vi "clone.vi"(0 "reference":refnum<class "SegmentedLineEdge.lvclass">, 5 "error in (no error)":errorcluster) -> (14 "reference out":refnum<class "SegmentedLineEdge.lvclass">, 15 "clonedEdge":refnum<class "AbstractEdge.lvclass">, 19 "error out":errorcluster)   [LabVIEW 2020, in "SegmentedLineEdge.lvclass"]
doc: "clone"
uses:
  <resource>/Framework/Providers/Open_GDS/UML/SegmentedLineEdge_class/SegmentedLineEdge.lvclass
  C:/Program Files (x86)/National Instruments/LabVIEW 2020/resource/Framework/Providers/Open_GDS/UML/GeneralPathEdge_class/GeneralPathEdge.lvclass
  C:/Program Files (x86)/National Instruments/LabVIEW 2020/resource/Framework/Providers/Open_GDS/UML/AbstractEdge_class/AbstractEdge.lvclass
  <resource>/Framework/Providers/Open_GDS/UML/AbstractEdge_class/AbstractEdge.lvclass
  <resource>/Framework/Providers/Open_GDS/UML/GeneralPathEdge_class/GeneralPathEdge.lvclass
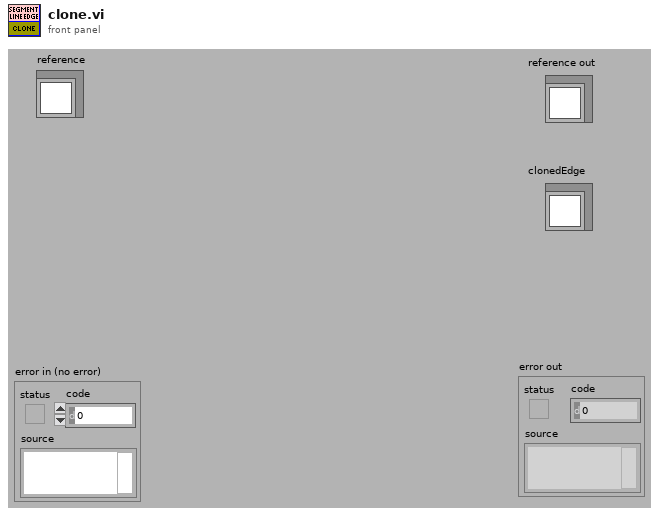
[diagram p1: front panel]
types:
  T1 = typedef "SegmentedLineEdge.lvclass/ObjectAttributes.ctl" = cluster{"lineStyle":refnum<class "LineStyle.lvclass">, "startArrowHead":refnum<class "ArrowHead.lvclass">, "endArrowHead":refnum<class "ArrowHead.lvclass">, "startLabel":string, "midLabel":string, "endLabel":string, "MidLabelOffset":T2, "SplitWire":bool}
  T2 = typedef "Point Point2D.ctl" = cluster{"x":dbl, "y":dbl}
  T3 = typedef "GeneralPathEdge.lvclass/ObjectAttributes.ctl" = cluster{"None":bool}
  T4 = typedef "AbstractEdge.lvclass/ObjectAttributes.ctl" = cluster{"start":refnum<class "AbstractNode.lvclass">, "end":refnum<class "AbstractNode.lvclass">}
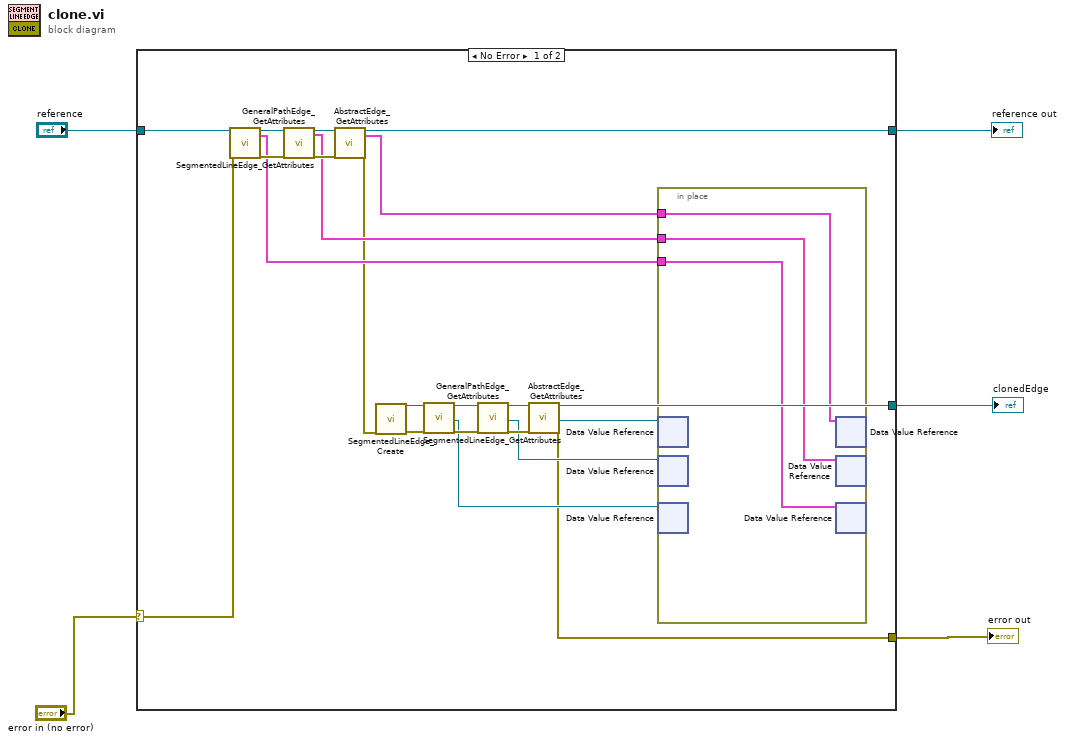
[diagram p0: block diagram]
diagram:
  n1 = case shown="No Error" "error in (no error)" {
    selector: "error in (no error)" -> [w13 w31]
    tunnel: "reference" -> [w9 w32]
    tunnel: [w7 w31] -> w4
    tunnel: [w8 w32] -> w3
    tunnel: [w6 _] -> w1
    frame No Error {
      n2 = call <resource>:"SegmentedLineEdge_GetAttributes.vi"("reference in"=w9, "error in (no error)"=w13) -> ("reference out"=w25:refnum<class "SegmentedLineEdge.lvclass">, "Data"=w19:T1, "error out"=w24:errorcluster)  [unwired: 1 in, 14 out]
      n3 = call <resource>:"GeneralPathEdge_GetAttributes.vi"("reference in"=w25, "error in (no error)"=w24) -> ("reference out"=w27:refnum<class "SegmentedLineEdge.lvclass">, "Data"=w18:T3, "error out"=w26:errorcluster)  [unwired: 14 in, 1 out]
      n4 = call <resource>:"AbstractEdge_GetAttributes.vi"("reference in"=w27, "error in (no error)"=w26) -> ("reference out"=w8:refnum<class "SegmentedLineEdge.lvclass">, "Data"=w17:T4, "error out"=w10:errorcluster)  [unwired: 14 in, 1 out]
      n5 = call <resource>:"SegmentedLineEdge_Create.vi"("error in (no error)"=w10) -> ("reference out"=w12:refnum<class "SegmentedLineEdge.lvclass">, "error out"=w11:errorcluster)  [unwired: 17 in]
      n6 = call <resource>:"SegmentedLineEdge_GetAttributes.vi"("reference in"=w12, "error in (no error)"=w11) -> ("reference out"=w22:refnum<class "SegmentedLineEdge.lvclass">, "DataRef"=w15:refnum<data-value>, "error out"=w23:errorcluster)  [unwired: 1 in, 14 out]
      n7 = call <resource>:"GeneralPathEdge_GetAttributes.vi"("reference in"=w22, "error in (no error)"=w23) -> ("reference out"=w20:refnum<class "SegmentedLineEdge.lvclass">, "DataRef"=w14:refnum<data-value>, "error out"=w21:errorcluster)  [unwired: 14 in, 1 out]
      n8 = call <resource>:"AbstractEdge_GetAttributes.vi"("reference in"=w20, "error in (no error)"=w21) -> ("reference out"=w6:refnum<class "SegmentedLineEdge.lvclass">, "DataRef"=w16:refnum<data-value>, "error out"=w7:errorcluster)  [unwired: 14 in, 1 out]
      n9 = in-place {
        in-place-border: w19 -> [w30]
        in-place-border: w18 -> [w29]
        in-place-border: w17 -> [w28]
        n10 = in-place-dvr #1(w16) -> ()  [unwired: 2 out]
        n11 = in-place-dvr #2(w14) -> ()  [unwired: 2 out]
        n12 = in-place-dvr #3(w15) -> ()  [unwired: 2 out]
        n13 = in-place-dvr #1(w28) -> ()  [unwired: 2 out]
        n14 = in-place-dvr #2(w29) -> ()  [unwired: 2 out]
        n15 = in-place-dvr #3(w30) -> ()  [unwired: 2 out]
      }
    }
    frame Error {
    }
  }
  "reference out" <- w3
  "error out" <- w4
  "clonedEdge" <- w1
